vi "move-REL-RAW.vi"(10 "Distance":dbl, 11 "Device in":refnum<k24>) -> (3 "Devicec out":refnum<k24>)   [LabVIEW 2014]
doc: "André Romero - 2019\nandretec@ifsc.usp.br"
uses:
  C:/users-lab/Andre/GITs/andretec/Thorlabs-Vector-Move/kinesisTec/Kinesis/Thorlabs.MotionControl.TCube.DCServoCLI.dll
  Kinesis/Thorlabs.MotionControl.TCube.DCServoCLI.dll
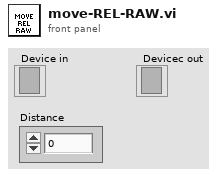
[diagram p1: front panel]
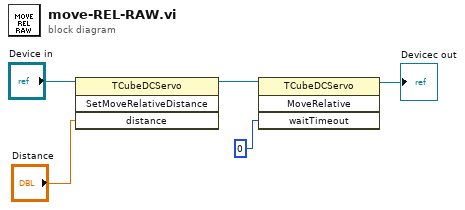
[diagram p0: block diagram]
diagram:
  n1 = invoke class="TCubeDCServo" method="SetMoveRelativeDistance"(reference="Device in", "distance"="Distance") -> (reference out=w1:refnum<k24>)  [unwired: 2 in, 3 out]
  n2 = invoke class="TCubeDCServo" method="MoveRelative"(reference=w1, "waitTimeout"=0) -> (reference out=→"Devicec out":refnum<k24>)  [unwired: 2 in, 3 out]
